vi "Scale Auto V.3.0.vi"() -> (3 "Stop":bool)   [LabVIEW 2017]
uses:
  Robot Global Data V.2.0.vi
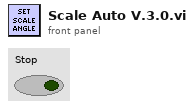
[diagram p1: front panel]
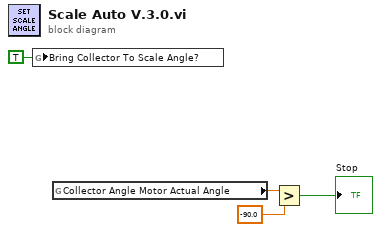
[diagram p0: block diagram]
diagram:
  n1 = global write "Robot Global Data V.2.0.vi" "Bring Collector To Scale Angle?"(TRUE ("Bring Collector To Scale Angle?")) -> ()
  n2 = global read "Robot Global Data V.2.0.vi" "Collector Angle Motor Actual Angle"() -> (w3:dbl)
  n3 = Greater?(x=w3, y=-90.0) -> (0:→"Stop":bool)
